vi "List Drivers.vi"(11 "error in (no error)":errorcluster) -> (15 "error out":errorcluster)   [LabVIEW 2021, in "Migrator.lvlib"]
uses:
  Migrator.lvlib
  <vilib>/Utility/traverseref.llb/TRef TravTarget.ctl
  <vilib>/Utility/traverseref.llb/VI Scripting - Traverse.lvlib
  Migrator Reusables/Migrator Reusables.lvlib
  Path Functions/Path Functions.lvlib
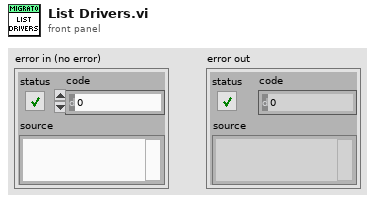
[diagram p1: front panel]
types:
  T1 = typedef "TRef TravTarget.ctl" = enum16{"FP", "BD", "Other"}
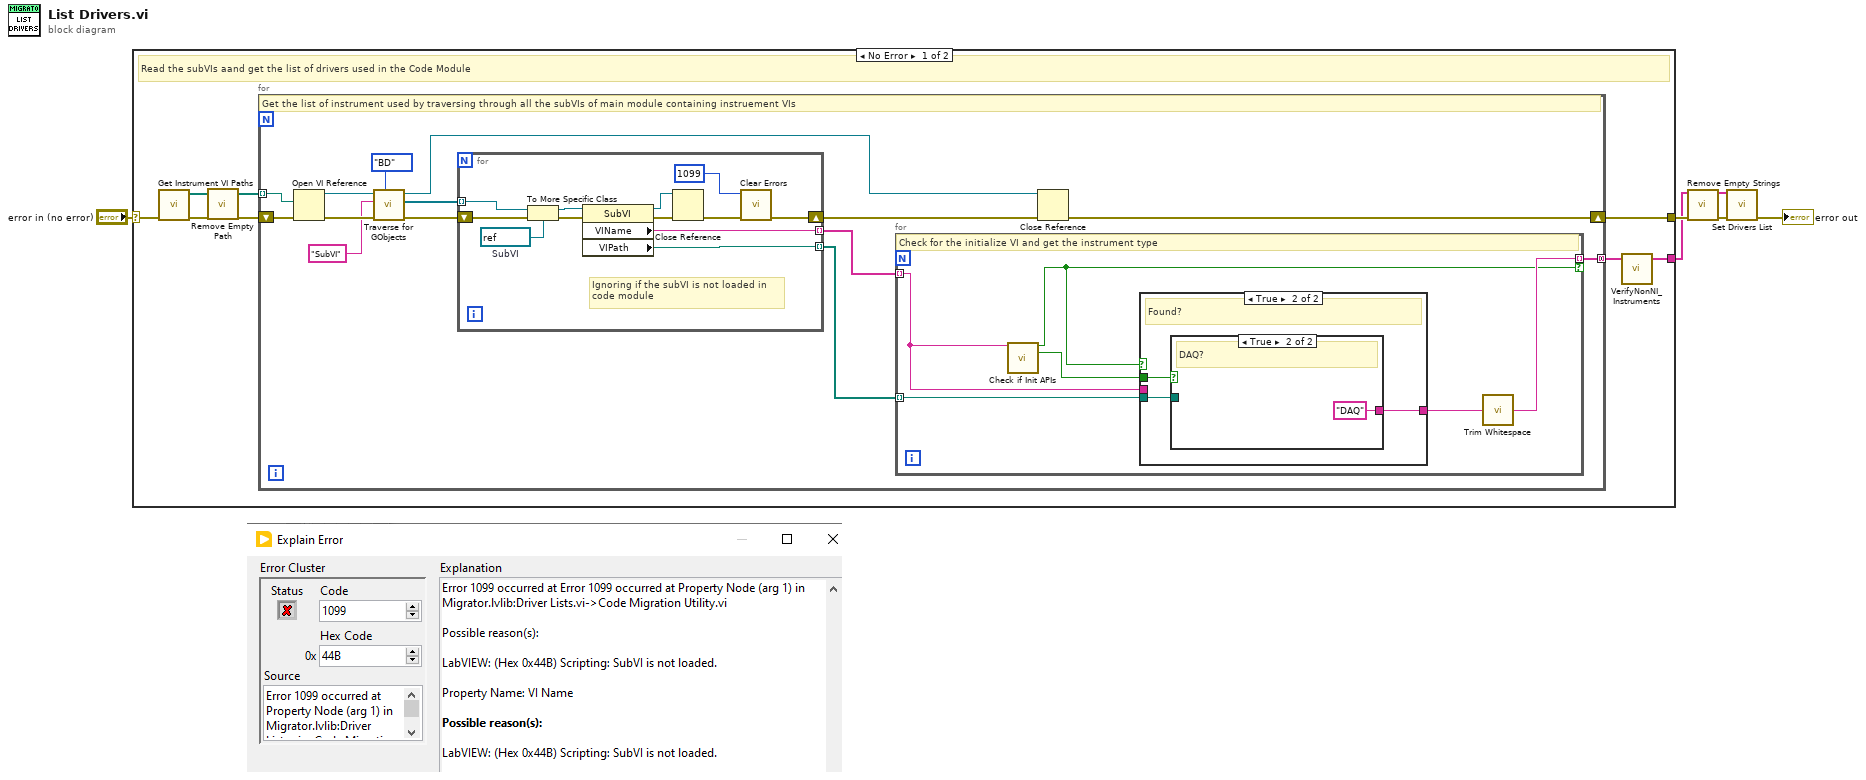
[diagram p0: block diagram]
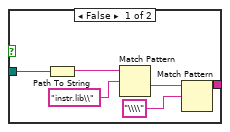
[diagram p3: hidden frame]
diagram:
  n1 = case shown="No Error" "error in (no error)" {
    selector: "error in (no error)" -> [w12 w55]
    tunnel: [w8 w55] -> w4
    tunnel: [w9 _] -> w2
    frame No Error {
      # "Read the subVIs aand get the list of drivers used in the Code Module"
      n2 = call "Get Instrument VI Paths.vi"("error in (no error)"=w12) -> ("error out"=w11:errorcluster, "Instr VI Paths[]"=w7:path[])  [unwired: 9 in]
      n3 = call "Remove Empty Path.vi"("Instr VI Paths in"=w7) -> ("Instr VI Paths out"=w6:path[])  [unwired: 4 in]
      n4 = for {
        tunnel: w6 -> [w21] mode=indexing
        tunnel: [w17] -> w10 mode=concatenating
        shift-right: [w15] -> w8
        shift-left: w11 -> [w20]
        # "Get the list of instrument used by traversing through all the subVIs of main module containing instruement VIs"
        n5 = Open VI Reference(vi path=w21, error in (no error)=w20) -> (vi reference=w16:refnum<vi>, error out=w24:errorcluster)  [unwired: 4 in]
        n6 = call <vilib>:"Traverse for GObjects.vi"("Traverse Target"=TRef_TravTarget."BD", "error in (no error)"=w24, "Class Name"="SubVI", "VI Refnum"=w16) -> ("error out"=w26:errorcluster, "References"=w25:refnum<vi>[], "dup VI Refnum"=w13:refnum<vi>)  [unwired: 4 in, 1 out]
        n7 = for {
          tunnel: w25 -> [w53] mode=indexing
          tunnel: [w49] -> w19 mode=indexing
          tunnel: [w48] -> w18 mode=indexing
          shift-right: [w44] -> w14
          shift-left: w26 -> [w52]
          w54 = refnum<vi> refnum  # SubVI
          # "Ignoring if the subVI is not loaded in\ncode module"
          n8 = To More Specific Class(target class=w54, reference=w53, error in=w52) -> (specific class reference=w51:refnum<vi>, error out=w50:errorcluster)
          n9 = property class="SubVI"(reference=w51, error in=w50) -> (reference out=w47:refnum<vi>, error out=w46:errorcluster, "VIName"=w49:string, "VIPath"=w48:path)
          n10 = Close Reference(reference=w47, error in (no error)=w46) -> (error out=w45:errorcluster)
          n11 = call <vilib>:"Clear Errors.vi"("error in (no error)"=w45, "specific error code to clear (0: all)"=1099) -> ("error out"=w44:errorcluster)  [unwired: 4 in, 1 out]
        }
        n12 = for {
          tunnel: w19 -> [w28] mode=indexing
          tunnel: w18 -> [w32] mode=indexing
          tunnel: [w31] -> w17 mode=indexing if=w29
          # "Check for the initialize VI and get the instrument type"
          n13 = call "Check if Init APIs.vi"("VIName"=w28) -> ("Instrument Driver Found?"=w29:bool, "DAQ?"=w27:bool)  [unwired: 13 in]
          n14 = case shown="True" w29 {
            tunnel: w32 -> [_ w35]
            tunnel: [_ w34] -> w30
            tunnel: w28 -> [_ _]
            tunnel: w27 -> [_ w33]
            frame False {
            }
            frame True {
              # "Found?"
              n15 = case shown="True" w33 {
                tunnel: w35 -> [w37 _]
                tunnel: [w36 "DAQ"] -> w34
                frame False {
                  n16 = Path To String(path=w37) -> (string=w38:string)
                  n17 = Match Pattern(string=w38, regular expression="instr.lib\\") -> (after substring=w40:string)  [unwired: 1 in, 3 out]
                  n18 = Match Pattern(string=w40, regular expression="\\\\") -> (before substring=w36:string)  [unwired: 1 in, 3 out]
                }
                frame True {
                  # "DAQ?"
                }
              }
            }
          }
          n19 = call <vilib>:"Trim Whitespace.vi"("string"=w30) -> ("trimmed string"=w31:string)  [unwired: 1 in]
        }
        n20 = Close Reference(reference=w13, error in (no error)=w14) -> (error out=w15:errorcluster)
      }
      n21 = call "VerifyNonNI_Instruments.vi"("Instrument Types In"=w10) -> ("Instrument Types Out"=w9:string[])  [unwired: 4 in]
    }
    frame Error {
    }
  }
  n22 = call "Remove Empty Strings.vi"("Instrument Types Out in"=w2) -> ("Instrument Types Out out"=w1:string[])  [unwired: 14 in]
  n23 = call "Set Drivers List.vi"("Name"=w1, "error in (no error)"=w4) -> ("error out"=→"error out":errorcluster)  [unwired: 13 in]
